vi "Configure IF Bandwith.vi"(8 "error in (no error)":errorcluster, 10 "IF BW [Hz]":dbl, 11 "VNA-FieldFox in":refnum<class "VNA-FieldFox.lvclass">) -> (0 "error out":errorcluster, 2 "IF BW used [Hz]":dbl, 3 "VNA-FieldFox out":refnum<class "VNA-FieldFox.lvclass">)   [LabVIEW 2020, in "VNA-FieldFox.lvclass"]
doc: "Configures the Intermidiate Frequency Bandwidth. \nIt chooses the closest supported bandwidth.\nIt returns the used IF BW."
uses:
  VNA-FieldFox.lvclass
  C:/Sandbox/Git_Sandbox/WiSpry Test Framework source code (LV20)/WiSpry Test Framework/Instruments/Instrument.lvclass
  C:/Sandbox/Git_Sandbox/WiSpry Test Framework source code (LV20)/WiSpry Test Framework/Instruments/Vector Network Analyzer/Vector Network Analyzer.lvclass
  Instrument.lvclass/Instrument.ctl
  Vector Network Analyzer.lvclass/Vector Network Analyzer.ctl
  Instrument.lvclass
  Vector Network Analyzer.lvclass
  <instrlib>/Agilent N99XX Series/Agilent N99XX Series.lvlib
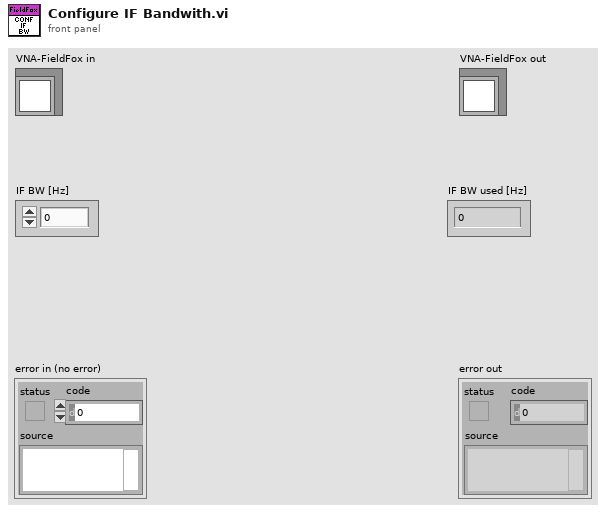
[diagram p1: front panel]
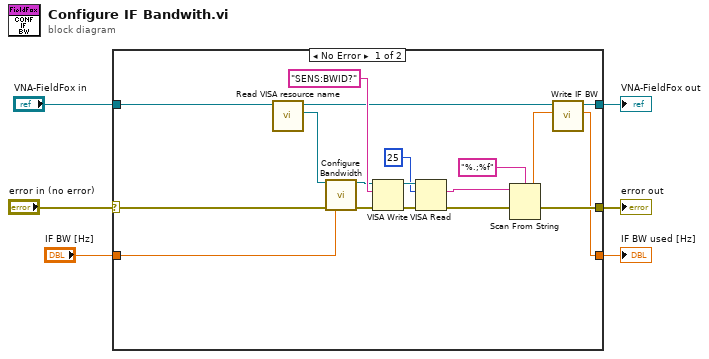
[diagram p0: block diagram]
diagram:
  n1 = case shown="No Error" "error in (no error)" {
    selector: "error in (no error)" -> [w14 w25]
    tunnel: "IF BW [Hz]" -> [w7 w26]
    tunnel: "VNA-FieldFox in" -> [w21 w24]
    tunnel: [w18 w24] -> w4
    tunnel: [w13 w25] -> w2
    tunnel: [w11 w26] -> w1
    frame No Error {
      n2 = call "Read VISA resource name.vi"("Instrument in"=w21) -> ("VISA resource name"=w10:refnum<visa-resource-name>, "Instrument out"=w15:refnum<class "VNA-FieldFox.lvclass">)  [unwired: 9 in]
      n3 = call <instrlib>:"Configure Bandwidth.vi"("VISA resource name"=w10, "error in (no error)"=w14, "IF Bandwidth (30000 Hz)"=w7) -> ("VISA resource name out"=w9:refnum<visa-resource-name>, "error out"=w8:errorcluster)  [unwired: 11 in]
      n4 = VISA Write(VISA resource name=w9, write buffer="SENS:BWID?", error in (no error)=w8) -> (VISA resource name out=w23:refnum<visa-resource-name>, error out=w20:errorcluster)  [unwired: 1 out]
      n5 = VISA Read(VISA resource name=w23, byte count=u32 25, error in (no error)=w20) -> (read buffer=w16:string, error out=w12:errorcluster)  [unwired: 2 out]
      n6 = Scan From String(format string="%.;%f", input string=w16, error in=w12) -> (error out=w13:errorcluster, output 1=w11:dbl)  [unwired: 2 in, 2 out]
      n7 = call "Write IF BW.vi"("IF BW"=w11, "Vector Network Analyzer in"=w15) -> ("Vector Network Analyzer out"=w18:refnum<class "VNA-FieldFox.lvclass">)  [unwired: 9 in]
    }
    frame Error {
    }
  }
  "error out" <- w2
  "VNA-FieldFox out" <- w4
  "IF BW used [Hz]" <- w1
